vi "启动参数设置.vi"() -> ()   [LabVIEW 2016, in "斯坦道总磷总氮V2.lvlib"]
panel:
  in  "关闭":bool
  in  "保存":bool
  out "启动队列名称":cluster{"String":string, "Value":u16}[](array[cluster])
  out "启动参数":string
  in  "氨氮":bool
  in  "总氮":bool
  in  "总磷":bool
  # "请选择要启动的参数"
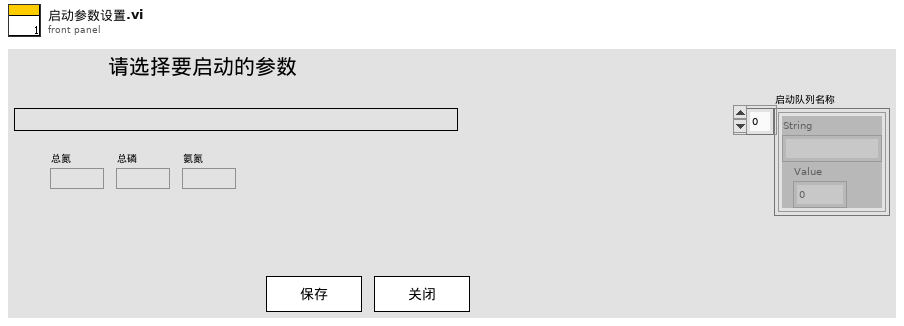
[diagram p1: front panel]
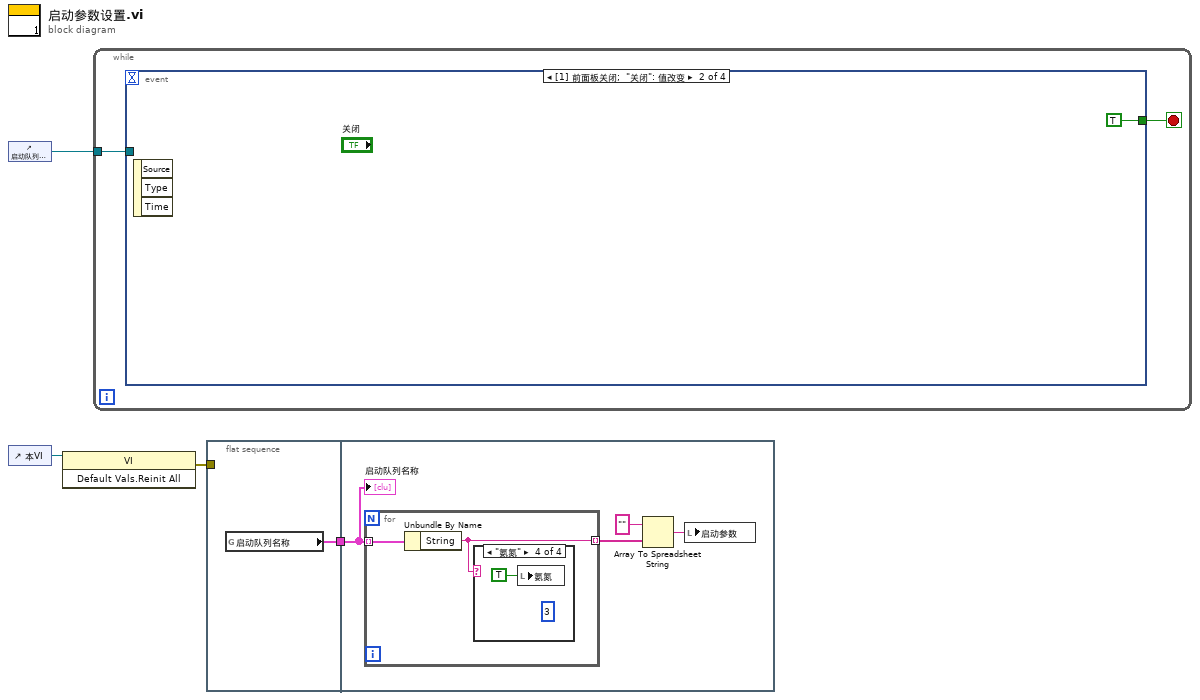
[diagram p0: block diagram]
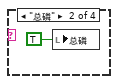
[diagram p3: hidden frame]
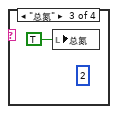
[diagram p4: hidden frame]
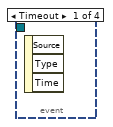
[diagram p5: hidden frame]
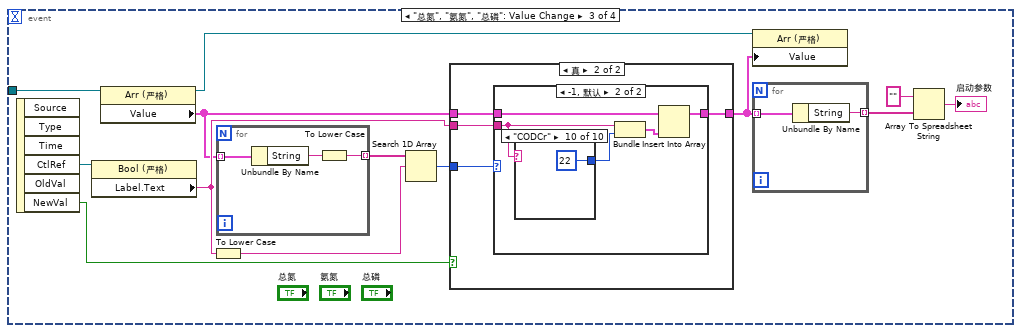
[diagram p6: hidden frame]
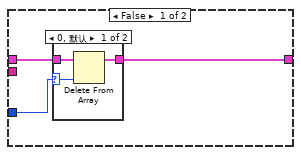
[diagram p7: hidden frame]
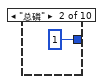
[diagram p11: hidden frame]
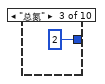
[diagram p12: hidden frame]
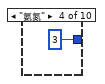
[diagram p13: hidden frame]
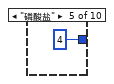
[diagram p14: hidden frame]
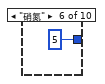
[diagram p15: hidden frame]
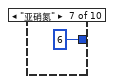
[diagram p16: hidden frame]
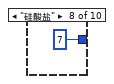
[diagram p17: hidden frame]
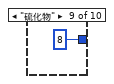
[diagram p18: hidden frame]
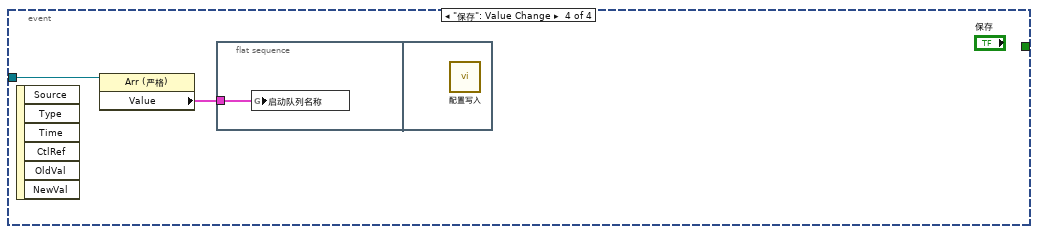
[diagram p19: hidden frame]
diagram:
  n1 = control-ref of="启动队列名称"() -> (w4:refnum<vi>)
  n2 = control-ref of="本VI"() -> (w3:refnum<vi>)
  n3 = invoke class="VI" method="Default Vals.Reinit All"(reference=w3) -> (error out=w2:errorcluster)  [unwired: 2 in, 2 out]
  n4 = while {
    tunnel: w4 -> [w5]
    stop <- w6 stop-if-true
    n5 = event shown="[1] 前面板关闭;  \"关闭\": 值改变" {
      selector: _ -> [_ _ _ _]
      dyn-events: _ -> [_ _ _ _]
      timeout: _ -> [_ _ _ _]
      tunnel: [_ TRUE _ _] -> w6
      tunnel: w5 -> [_ _ w12 w53]
      event Timeout {
        n6 = event-data() -> ()  [unwired: 1 in, 3 out]
      }
      event Panel Close; "关闭": Value Change {
        n7 = event-data() -> ()  [unwired: 1 in, 3 out]
      }
      event "总氮", "氨氮", "总磷": Value Change {
        n8 = event-data() -> ("CtlRef"=w20:refnum<vi>, "NewVal"=w19:bool)  [unwired: 1 in, 4 out]
        n9 = property class="Bool (严格)"(reference=w20) -> ("Label.Text"=w17:string)  [unwired: 1 in, 2 out]
        n10 = property class="Arr (严格)"(reference=w12) -> (reference out=w10:refnum<vi>, "Value"=w11:cluster{"String":string, "Value":u16}[])  [unwired: 1 in, 1 out]
        n11 = To Lower Case(string=w17) -> (all lower case string=w8:string)
        n12 = for {
          tunnel: w11 -> [w25] mode=indexing
          tunnel: [w23] -> w18 mode=indexing
          n13 = Unbundle By Name(w25) -> ("String"=w24:string)
          n14 = To Lower Case(string=w24) -> (all lower case string=w23:string)
        }
        n15 = Search 1D Array(1D array=w18, element=w8) -> (index of element=w16:i32)  [unwired: 1 in]
        n16 = case shown="真" w19 {
          tunnel: w17 -> [_ w35]
          tunnel: w11 -> [w27 w36]
          tunnel: w16 -> [w28 w34]
          tunnel: [w26 w33] -> w9
          frame False {
            n17 = case shown="0, 默认" w28 {
              selector: w28 -> [w30 _]
              tunnel: w27 -> [w31 w32]
              tunnel: [w29 w32] -> w26
              frame 0, Default {
                n18 = Delete From Array(array=w31, index=w30) -> (array with subset deleted=w29:cluster{"String":string, "Value":u16}[])  [unwired: 1 in, 1 out]
              }
              frame -1 {
              }
            }
          }
          frame True {
            n19 = case shown="-1, 默认" w34 {
              tunnel: w36 -> [w37 w42]
              tunnel: w35 -> [_ w41]
              tunnel: [w37 w38] -> w33
              frame 0 {
              }
              frame -1, Default {
                n20 = case shown="\"CODCr\"" w41 {
                  tunnel: [_ 1 2 3 4 5 6 7 8 22] -> w40
                  frame Default {
                  }
                  frame "总磷" {
                  }
                  frame "总氮" {
                  }
                  frame "氨氮" {
                  }
                  frame "磷酸盐" {
                  }
                  frame "硝氮" {
                  }
                  frame "亚硝氮" {
                  }
                  frame "硅酸盐" {
                  }
                  frame "硫化物" {
                  }
                  frame "CODCr" {
                  }
                }
                n21 = Bundle("Label.Text"=w41, w40) -> (w39:cluster{"Label.Text":string, i32})  [unwired: 1 in]
                n22 = Insert Into Array(array=w42, new element=w39) -> (w38:cluster{"String":string, "Value":u16}[])  [unwired: 1 in]
              }
            }
          }
        }
        n23 = property class="Arr (严格)"(reference=w10, "Value"=w9) -> ()  [unwired: 1 in, 2 out]
        n24 = for {
          tunnel: w9 -> [w22] mode=indexing
          tunnel: [w21] -> w15 mode=indexing
          n25 = Unbundle By Name(w22) -> ("String"=w21:string)
        }
        n26 = Array To Spreadsheet String(array=w15, 3:"" ("格式字符串")) -> (spreadsheet string=→"启动参数":string)  [unwired: 1 in]
      }
      event "保存": Value Change {
        n27 = event-data() -> ()  [unwired: 1 in, 6 out]
        n28 = property class="Arr (严格)"(reference=w53) -> ("Value"=w52:cluster{"String":string, "Value":u16}[])  [unwired: 1 in, 2 out]
        n29 = flat-sequence {
          tunnel: w52 -> [w54]
          frame #0 {
            n30 = global write "总磷总氮断电保存全局变量.vi" "启动队列名称"(w54) -> ()
          }
          frame #1 {
            n31 = call "配置写入.vi"() -> ()  [unwired: 11 in, 1 out]
          }
        }
      }
    }
  }
  n32 = flat-sequence {
    tunnel: w2 -> [_]
    tunnel: [w55] -> w1
    tunnel: w1 -> [w56]
    frame #0 {
      n33 = global read "总磷总氮断电保存全局变量.vi" "启动队列名称"() -> (w55:cluster{"String":string, "Value":u16}[])
    }
    frame #1 {
      n34 = for {
        tunnel: w56 -> [w61] mode=indexing
        tunnel: [w60] -> w58 mode=indexing
        n35 = Unbundle By Name(w61) -> ("String"=w60:string)
        n36 = case shown="\"氨氮\"" w60 {
          frame Default {
          }
          frame "总磷" {
            n37 = local write "总磷"(TRUE ("总磷")) -> ()
          }
          frame "总氮" {
            (unwired) 2
            n38 = local write "总氮"(TRUE ("总磷")) -> ()
          }
          frame "氨氮" {
            (unwired) 3
            n39 = local write "氨氮"(TRUE ("总磷")) -> ()
          }
        }
      }
      n40 = Array To Spreadsheet String(array=w58, 3:"" ("格式字符串")) -> (spreadsheet string=w57:string)  [unwired: 1 in]
      n41 = local write "启动参数"(w57) -> ()
      "启动队列名称" <- w56
    }
  }
